vi "Kaelus PIM Set MeasBand.vi"(7 "Comm Interface":T1, 8 "error in (no error)":errorcluster, 11 "Stimulus":T2={"Carrier Frequencies"={"C1 Freq, MHz"=0.0, "C2 Freq, MHz"=0.0}, "Carrier Powers"={"C1 Power,dBm"=0.0, "C2 Power, dBm"=0.0}, "Measurement Parameters"={"IM Order"=0, "Averaging"=1, "Direction"=0, "Enable ALC?"=FALSE, "Enable SingleIM?"=FALSE, "Display Units"=enum."dBm", "VA Hold?"=FALSE, "DUT PORT"=enum."Port 1"}, "Measurement Setup"={"Meas Type"=enum."Time", "TXStep"=0}} {"Measurement Setup"."TXStep" items=[".2", ".4", "1.0", "2.0"]; "Measurement Parameters"."Direction" items=["Reverse", "Forward", "Auxiliary"]; "Measurement Parameters"."IM Order" items=["3rd", "5th", "7th", "9th", "11th", "13th", "15th", "17th", "19th", "21st", "23rd", "25th", "27th", "29th", "31st", "33rd"]; "Measurement Parameters"."Averaging" items=["None", "Minimum", "Normal", "High", "Maximum"]}) -> (0 "error out":errorcluster)   [LabVIEW 2011]
uses:
  PIM Stimulus.ctl
  PIM Cmd Params.ctl
  BPIMCore EXT/HW IO/IMOrder.ctl
  BPIMCore EXT/HW IO/HW Averaging.ctl
  BPIMCore EXT/HW IO/MeasMode.ctl
  BPIMCore EXT/Display/display_unit_format.ctl
  BPIMCore EXT/HW IO/DUTport.ctl
  BPIMCore EXT/HW IO/PIM Sweep Step Size.ctl
  PIM Interface Language.ctl
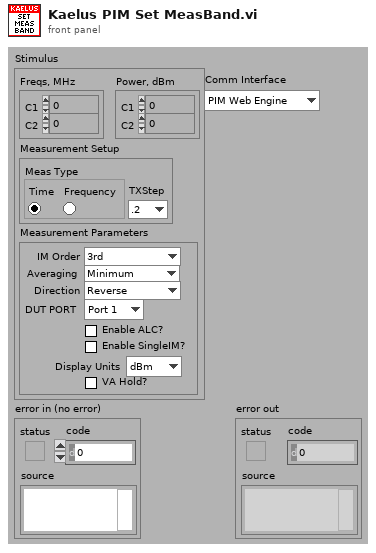
[diagram p1: front panel]
types:
  T1 = typedef "PIM Interface Language.ctl" = enum16{"PIM Web Engine", "PIM HW Engine"}
  T2 = typedef "PIM Stimulus.ctl" = cluster{"Carrier Frequencies":cluster{"C1 Freq, MHz":dbl, "C2 Freq, MHz":dbl}, "Carrier Powers":cluster{"C1 Power,dBm":dbl, "C2 Power, dBm":dbl}, "Measurement Parameters":T3, "Measurement Setup":cluster{"Meas Type":enum32{"Time", "Frequency"}, "TXStep":T9}}
  T3 = typedef "PIM Cmd Params.ctl" = cluster{"IM Order":T4, "Averaging":T5, "Direction":T6, "Enable ALC?":bool, "Enable SingleIM?":bool, "Display Units":T7, "VA Hold?":bool, "DUT PORT":T8}
  T4 = typedef "IMOrder.ctl" = u8
  T5 = typedef "HW Averaging.ctl" = u16
  T6 = typedef "MeasMode.ctl" = u16
  T7 = typedef "display_unit_format.ctl" = enum16{"dBm", "dBc"}
  T8 = typedef "DUTport.ctl" = enum16{"Port 1", "Port 2"}
  T9 = typedef "PIM Sweep Step Size.ctl" = u16
  T10 = typedef "Test Set Definition.ctl" = cluster{"General":cluster{"ID":u32, "Model":string, "Dual Port?":bool, "Options":string, "Options":cluster{"E":bool, "K":bool, "H":bool, "W":bool, "F":bool}, "Cal File":path}, "Receiver":cluster{"Fstart, MHz":dbl, "Fstop MHz":dbl, "Fstep MHz":dbl, "IF, MHz":dbl}, "RX Band":cluster{"Fstart, MHz":dbl, "Fstop MHz":dbl}, "TX 1":cluster{"Fstart, MHz":dbl, "Fstop MHz":dbl, "Pmax, dBm":dbl, "Pstep, dB":dbl}, "TX 2":cluster{"Fstart, MHz":dbl, "Fstop MHz":dbl, "Pmax, dBm":dbl, "Pstep, dB":dbl}, "Low-side?":bool}
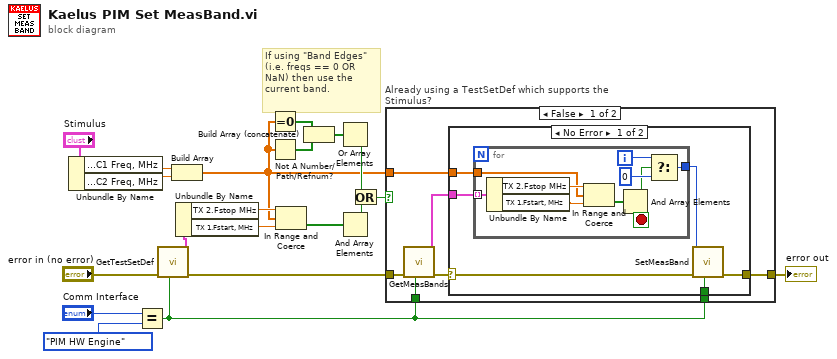
[diagram p0: block diagram]
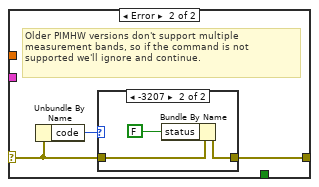
[diagram p2: hidden frame]
diagram:
  # "If using \"Band Edges\" (i.e. freqs == 0 OR NaN) then use the current band."
  n1 = Unbundle By Name("Stimulus") -> ("Carrier Frequencies.C1 Freq, MHz"=w19:dbl, "Carrier Frequencies.C2 Freq, MHz"=w18:dbl)
  n2 = Equal?(x="Comm Interface", y=PIM_Interface_Language."PIM HW Engine" ("Interface")) -> (x = y?=w1:bool)
  n3 = call "GetTestSetDef.vi"("Legacy (f)?"=w1, "error in (no error)"="error in (no error)") -> ("error out"=w16:errorcluster, "TestSetDef"=w14:T10)  [unwired: 8 out]
  n4 = Build Array(w19, w18) -> (w7:dbl[])
  n5 = Unbundle By Name(w14) -> ("TX 2.Fstop MHz"=w13:dbl, "TX 1.Fstart, MHz"=w12:dbl)
  n6 = Equal To 0?(x=w7) -> (x = 0?=w6:bool[])
  n7 = Not A Number/Path/Refnum?(number/path/refnum=w7) -> (NaN/Path/Refnum?=w5:bool[])
  n8 = In Range and Coerce(upper limit=w13, x=w7, lower limit=w12) -> (In Range?=w11:bool[])  [unwired: 1 out]
  n9 = Build Array (concatenate)(w6, w5) -> (w4:bool[])
  n10 = Or Array Elements(Boolean array=w4) -> (logical OR=w9:bool)
  n11 = And Array Elements(Boolean array=w11) -> (logical AND=w10:bool)
  n12 = Or(x=w9, y=w10) -> (x .or. y?=w8:bool)
  n13 = case "Already using a TestSetDef which supports the Stimulus?" shown="False" w8 {
    tunnel: w16 -> [w26 w50]
    tunnel: [w25 w50] -> w15
    tunnel: w7 -> [w24 _]
    tunnel: w1 -> [w22 _]
    tunnel: w1 -> [w21 _]
    frame False {
      n14 = call "GetMeasBands.vi"("Legacy (f)?"=w22, "error in (no error)"=w26) -> ("error out"=w23:errorcluster, "TestSets"=w27:T10[])  [unwired: 8 out]
      n15 = case shown="No Error" w23 {
        selector: w23 -> [w29 w43]
        tunnel: w27 -> [w33 _]
        tunnel: [w31 w45] -> w25
        tunnel: w24 -> [w30 _]
        tunnel: w21 -> [w28 _]
        frame No Error {
          n16 = for {
            tunnel: w33 -> [w36] mode=indexing
            tunnel: w30 -> [w40]
            tunnel: [w34] -> w32
            i -> [w39]
            stop <- w35 stop-if-true
            n17 = Unbundle By Name(w36) -> ("TX 2.Fstop MHz"=w42:dbl, "TX 1.Fstart, MHz"=w41:dbl)
            n18 = In Range and Coerce(upper limit=w42, x=w40, lower limit=w41) -> (In Range?=w38:bool[])  [unwired: 1 out]
            n19 = And Array Elements(Boolean array=w38) -> (logical AND=w35:bool)
            n20 = Select(t=w39, s=w35, f=0) -> (s? t:f=w34:i32)
          }
          n21 = call "SetMeasBand.vi"("Legacy (f)?"=w28, "error in (no error)"=w29, "Band Index"=w32) -> ("error out"=w31:errorcluster)  [unwired: 8 out]
        }
        frame Error {
          # "Older PIMHW versions don't support multiple measurement bands, so if the command is not supported we'll ignore and continue."
          n22 = Unbundle By Name(w43) -> ("code"=w44:i32)
          n23 = case shown="-3207" w44 {
            tunnel: w43 -> [w46 w49]
            tunnel: [w46 w48] -> w45
            frame 0, Default {
            }
            frame -3207 {
              n24 = Bundle By Name(cluster=w49, "status"=FALSE) -> (w48:errorcluster)
            }
          }
        }
      }
    }
    frame True {
    }
  }
  "error out" <- w15
